vi "Extract FFT of Real Sequence from FFT Output.vi"(7 "FFT Size":T1=enum."8192", 8 "Input Valid":bool, 11 "Input X(k)":fxp<+,64,64>) -> (0 "Output Valid":bool, 2 "X(N-k)":fxp<+,64,64>, 3 "X(k)":fxp<+,64,64>)   [LabVIEW 2011]
doc: "<b> Latency = 6 Ticks </b>"
uses:
  <userlib>/FPGA Library/Code Development/Signal Processing/FFT Block/FFT/FFT Size.ctl
  <vilib>/rvi/FXPMathLib/basic elements/FxpDiscreteDelay/XNode/nifxpmath_DiscreteDelay.xnode
  <instrlib>/FlexRIO/Libraries/Helper VIs/NI FlexRIO Helper VIs.lvlib
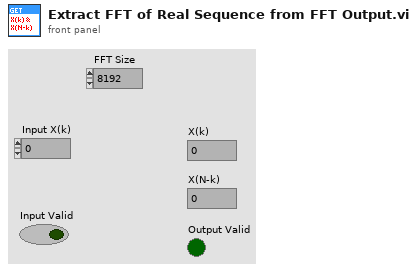
[diagram p1: front panel]
types:
  T1 = typedef "FFT Size.ctl" = enum16{"32", "64", "128", "256", "512", "1024", "2048", "4096", "8192", "16384", "32768", "65536"}
  T2 = typedef "BRAM State.ctl" = enum8{"Write to Bank", "Read from Bank"}
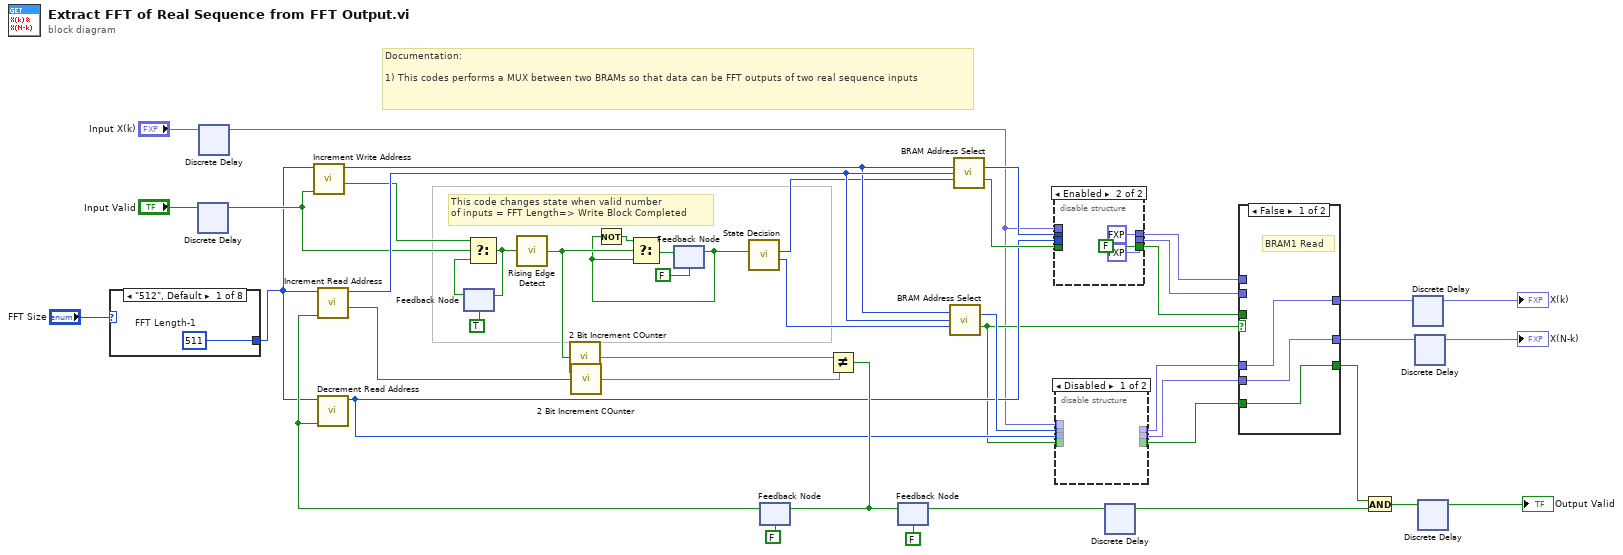
[diagram p0: block diagram]
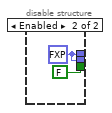
[diagram p2: hidden frame]
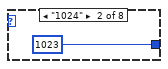
[diagram p4: hidden frame]
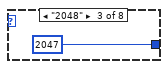
[diagram p5: hidden frame]
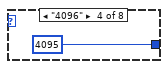
[diagram p6: hidden frame]
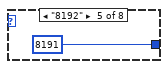
[diagram p7: hidden frame]
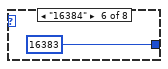
[diagram p8: hidden frame]
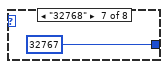
[diagram p9: hidden frame]
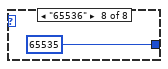
[diagram p10: hidden frame]
diagram:
  # "This code changes state when valid number\nof inputs = FFT Length=> Write Block Completed"
  # "Documentation:\n\n1) This codes performs a MUX between two BRAMs so that data can be FFT outputs of two real sequence inputs"
  n1 = case shown="\"512\", Default" "FFT Size" {
    tunnel: [w47 u16 1023 u16 2047 u16 4095 u16 8191 u16 16383 u16 32767 u16 65535 ("FFT Length-1")] -> w1
    frame "512", Default {
      w47 = u16 511  # FFT Length-1
    }
    frame "1024" {
    }
    frame "2048" {
    }
    frame "4096" {
    }
    frame "8192" {
    }
    frame "16384" {
    }
    frame "32768" {
    }
    frame "65536" {
    }
  }
  n2 = xnode "Discrete Delay"("D"="Input Valid") -> ("Q"=w6:bool)
  n3 = xnode "Discrete Delay"("D"="Input X(k)") -> ("Q"=w7:fxp<+,64,64>)
  n4 = call <userlib>:"Increment Write Address.vi"("INC?"=w6, "rollover"=w1) -> ("roll over"=w38:bool, "count"=w41:u16)  [unwired: 7 in, 1 out]
  n5 = feedback #1(TRUE ("roll over")) -> (w37:bool)
  n6 = Select(t=w38, s=w6, f=w37) -> (s? t:f=w36:bool)
  n7 = feedback-in #1(w36) -> ()
  n8 = call <instrlib>:"Rising Edge Detect.vi"("signal"=w36) -> ("edge detected"=w39:bool)  [unwired: 14 in]
  n9 = call <userlib>:"2 Bit Increment COunter.vi"("Increment"=w39) -> ("Counter Value"=w44:fxp<+,3,3>)  [unwired: 14 in]
  n10 = feedback #2(FALSE) -> (w18:bool)
  n11 = Not(x=w18) -> (.not. x?=w40:bool)
  n12 = Select(t=w40, s=w39, f=w18) -> (s? t:f=w34:bool)
  n13 = feedback-in #2(w34) -> ()
  n14 = call <userlib>:"State Decision.vi"("Change?"=w18) -> ("BRAM1 State"=w20:T2, "BRAM0 State"=w32:T2)  [unwired: 9 in]
  n15 = feedback #3(FALSE) -> (w31:bool)
  n16 = call <userlib>:"Increment Read Address.vi"("INC?"=w31, "rollover"=w1) -> ("roll over"=w45:bool, "count"=w46:u16)  [unwired: 8 in]
  n17 = call <userlib>:"Decrement Read Address.vi"("DEC?"=w31, "Load Value"=w1) -> ("count"=w22:u16)  [unwired: 8 in, 1 out]
  n18 = call <userlib>:"2 Bit Increment COunter.vi"("Increment"=w45) -> ("Counter Value"=w42:fxp<+,3,3>)  [unwired: 14 in]
  n19 = Not Equal?(x=w44, y=w42) -> (x != y?=w30:bool)
  n20 = feedback-in #3(w30) -> ()
  n21 = feedback #4(FALSE) -> (w29:bool)
  n22 = feedback-in #4(w30) -> ()
  n23 = call <userlib>:"BRAM Address Select.vi"("Write Address"=w41, "Read Address"=w46, "Read/Write?"=w20) -> ("BRAM Address"=w23:u16, "Write?"=w17:bool)  [unwired: 11 in]
  n24 = call <userlib>:"BRAM Address Select.vi"("Write Address"=w41, "Read Address"=w46, "Read/Write?"=w32) -> ("BRAM Address"=w26:u16, "Write?"=w25:bool)  [unwired: 11 in]
  n25 = disable-structure shown="Enabled" {
    disable-tunnel: w26 -> [_ _]
    disable-tunnel: w25 -> [_ _]
    disable-tunnel: w22 -> [_ _]
    disable-tunnel: [_ fxp<+,64,64> 0.0 ("Data from Address 1")] -> w14
    disable-tunnel: [_ fxp<+,64,64> 0.0 ("Data from Address 2")] -> w13
    disable-tunnel: [_ FALSE ("Data Valid")] -> w12
    disable-tunnel: w7 -> [_ _]
    frame Disabled {
    }
    frame Enabled {
    }
  }
  n26 = disable-structure shown="Disabled" {
    disable-tunnel: w23 -> [_ _]
    disable-tunnel: w22 -> [_ _]
    disable-tunnel: w17 -> [_ _]
    disable-tunnel: [_ w59] -> w16
    disable-tunnel: [_ w59] -> w15
    disable-tunnel: [_ FALSE ("Data Valid")] -> w11
    disable-tunnel: w7 -> [_ _]
    frame Disabled {
    }
    frame Enabled {
      w59 = fxp<+,64,64> 0.0 ("Data from Address 1")
    }
  }
  n27 = xnode "Discrete Delay"("D"=w29) -> ("Q"=w19:bool)
  n28 = case shown="False" w17 {
    tunnel: w16 -> [w62 _]
    tunnel: [w62 w65] -> w9
    tunnel: w15 -> [w61 _]
    tunnel: [w61 w64] -> w8
    tunnel: w14 -> [_ w65]
    tunnel: w13 -> [_ w64]
    tunnel: w12 -> [_ w63]
    tunnel: [w60 w63] -> w10
    tunnel: w11 -> [w60 _]
    frame False {
      # "BRAM1 Read"
    }
    frame True {
    }
  }
  n29 = And(x=w10, y=w19) -> (x .and. y?=w27:bool)
  n30 = xnode "Discrete Delay"("D"=w9) -> ("Q"=→"X(k)":fxp<+,64,64>)
  n31 = xnode "Discrete Delay"("D"=w8) -> ("Q"=→"X(N-k)":fxp<+,64,64>)
  n32 = xnode "Discrete Delay"("D"=w27) -> ("Q"=→"Output Valid":bool)
